vi "create.vi"(8 "error in":errorcluster, 10 "parent":refnum<class "identifying queue.lvclass">, 11 "uninitialized communicator":refnum<class "communicator.lvclass">) -> (0 "error out":errorcluster, 3 "communicator out":refnum<class "communicator.lvclass">)   [LabVIEW 2015, in "communicator.lvclass"]
uses:
  communicator.lvclass
  communicator queue/identifying queue.lvclass
  communicator.lvclass/communicator.ctl
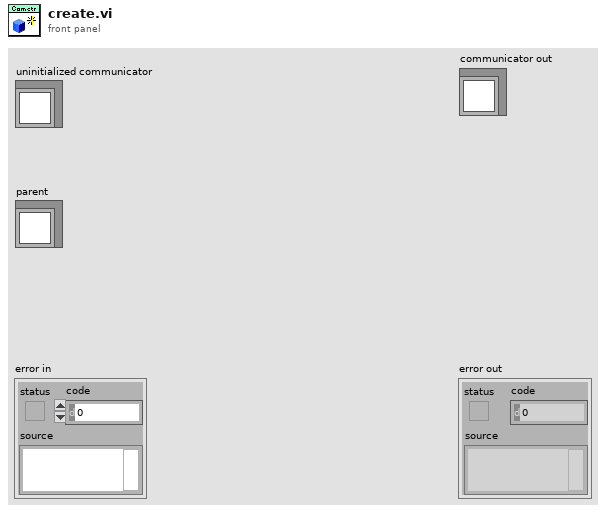
[diagram p1: front panel]
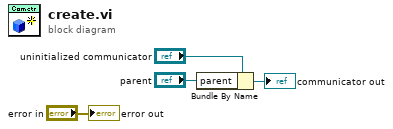
[diagram p0: block diagram]
diagram:
  n1 = Bundle By Name(cluster="uninitialized communicator", "parent"="parent") -> (→"communicator out":refnum<class "communicator.lvclass">)
  "error out" <- "error in"
